vi "AB_1200_1100_Project_InteropAssembly_Info.vi"(7 "action":T3, 8 "error in (no error)":errorcluster, 10 "InteropAssebly info in":T2, 11 "Object In":T1) -> (0 "error out":errorcluster, 2 "InteropAssebly info out":T2, 3 "Object Out":T1)   [LabVIEW 2020]
uses:
  <vilib>/AppBuilder/RW_Project/AB_RW_Project_PropBag_Action.ctl
  <resource>/Framework/Providers/API/ItemRef.ctl
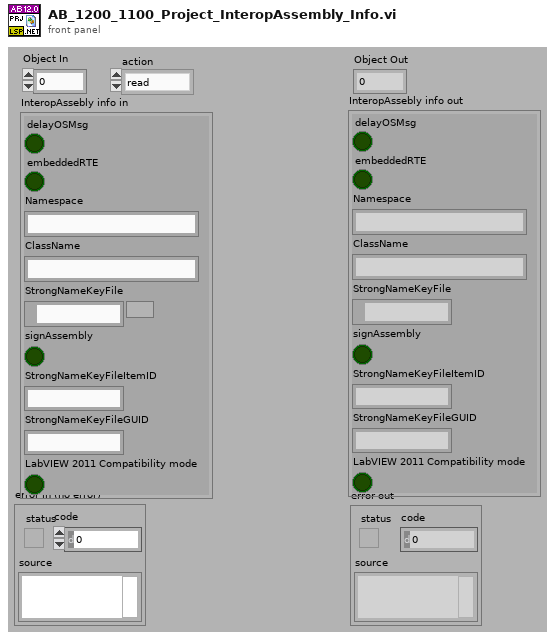
[diagram p1: front panel]
types:
  T1 = typedef "ItemRef.ctl" = u64
  T2 = cluster{"delayOSMsg":bool, "embeddedRTE":bool, "Namespace":string, "ClassName":string, "StrongNameKeyFile":path, "signAssembly":bool, "StrongNameKeyFileItemID":string, "StrongNameKeyFileGUID":string, "LabVIEW 2011 Compatibility mode":bool}
  T3 = typedef "AB_RW_Project_PropBag_Action.ctl" = enum16{"read", "write", "clear", "readPrevious", "writePrevious", "clearPrevious"}
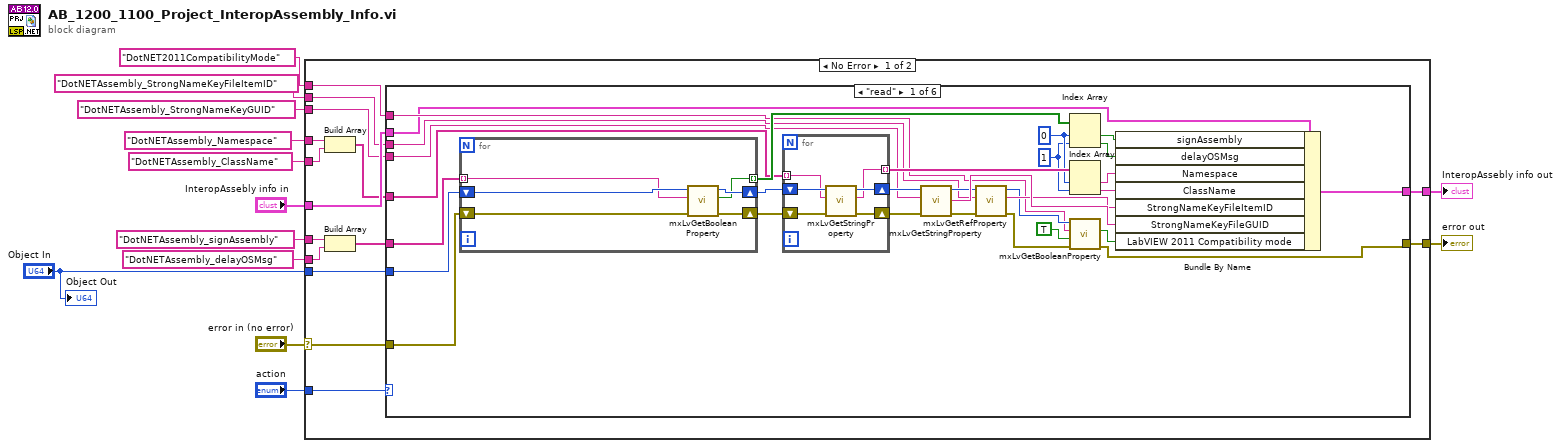
[diagram p0: block diagram]
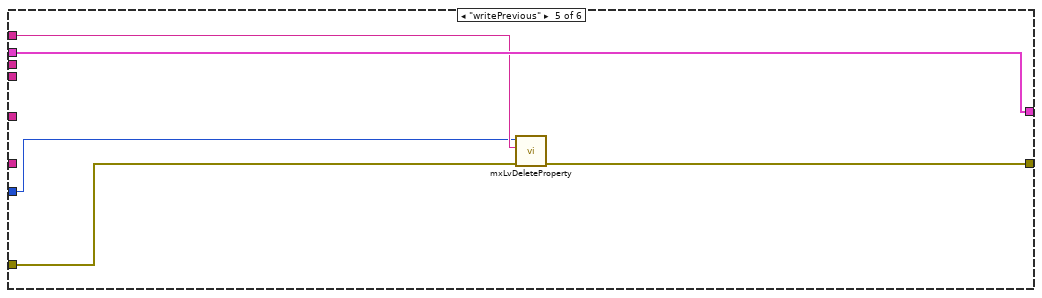
[diagram p5: hidden frame]
diagram:
  n1 = case shown="No Error" "error in (no error)" {
    selector: "error in (no error)" -> [w18 w85]
    tunnel: "Object In" -> [w27 _]
    tunnel: [w28 w84] -> w8
    tunnel: "InteropAssebly info in" -> [w26 w84]
    tunnel: "action" -> [w25 _]
    tunnel: "DotNETAssembly_Namespace" -> [w24 _]
    tunnel: "DotNETAssembly_ClassName" -> [w23 _]
    tunnel: "DotNETAssembly_StrongNameKeyGUID" -> [w21 _]
    tunnel: "DotNETAssembly_delayOSMsg" -> [w20 _]
    tunnel: [w17 w85] -> w4
    tunnel: "DotNETAssembly_StrongNameKeyFileItemID" -> [w16 _]
    tunnel: "DotNETAssembly_signAssembly" -> [w15 _]
    tunnel: "DotNET2011CompatibilityMode" -> [w14 _]
    frame No Error {
      n2 = Build Array(w24, w23) -> (w22:string[])
      n3 = Build Array(w15, w20) -> (w19:string[])
      n4 = case shown="\"read\"" w25 {
        tunnel: [w30 w72 w74 w76 w81 w83] -> w28
        tunnel: w27 -> [w37 _ _ _ w77 _]
        tunnel: w26 -> [w31 w72 w74 w76 w81 w83]
        tunnel: w22 -> [w35 _ _ _ _ _]
        tunnel: w21 -> [w34 _ _ _ _ _]
        tunnel: w19 -> [w36 _ _ _ _ _]
        tunnel: w18 -> [w38 w71 w73 w75 w79 w82]
        tunnel: [w29 w71 w73 w75 w78 w82] -> w17
        tunnel: w16 -> [w33 _ _ _ _ _]
        tunnel: w14 -> [w32 _ _ _ w80 _]
        frame "read" {
          w44 = 1 ("index")
          w52 = 0 ("index")
          n5 = for {
            shift-right: [w63] -> w55
            shift-left: w37 -> [w64]
            tunnel: w36 -> [w62] mode=indexing
            tunnel: [w61] -> w54 mode=indexing
            shift-right: [w59] -> w53
            shift-left: w38 -> [w60]
            n6 = call <resource>:"mxLvGetBooleanProperty.vi"("error in"=w60, "Tag"=w62, "Item"=w64) -> ("error out"=w59:errorcluster, "Value"=w61:bool, "Item"=w63:T1)  [unwired: 1 in, 5 out]
          }
          n7 = for {
            shift-right: [w69] -> w51
            shift-left: w55 -> [w70]
            tunnel: [w68] -> w58 mode=indexing
            tunnel: w35 -> [w67] mode=indexing
            shift-right: [w65] -> w50
            shift-left: w53 -> [w66]
            n8 = call <resource>:"mxLvGetStringProperty.vi"("Error In"=w66, "Tag"=w67, "Item"=w70) -> ("Error Out"=w65:errorcluster, "Value"=w68:string, "Item"=w69:T1)  [unwired: 6 out]
          }
          n9 = call <resource>:"mxLvGetStringProperty.vi"("Error In"=w50, "Tag"=w34, "Item"=w51) -> ("Error Out"=w47:errorcluster, "Value"=w49:string, "Item"=w46:T1)  [unwired: 6 out]
          n10 = call <resource>:"mxLvGetRefProperty.vi"("Error In"=w47, "Tag"=w33, "Item"=w46) -> ("Error Out"=w42:errorcluster, "Value"=w48:string, "Item"=w39:T1)  [unwired: 6 out]
          n11 = Index Array(array=w54, index #1=w52, index #2=w44) -> (element #1=w45:bool, element #2=w43:bool)
          n12 = Index Array(array=w58, index #1=w52, index #2=w44) -> (element #1=w57:string, element #2=w56:string)
          n13 = call <resource>:"mxLvGetBooleanProperty.vi"("error in"=w42, "Default Value (F)"=TRUE, "Tag"=w32, "Item"=w39) -> ("error out"=w29:errorcluster, "Value"=w41:bool)  [unwired: 6 out]
          n14 = Bundle By Name(cluster=w31, "signAssembly"=w45, "delayOSMsg"=w43, "Namespace"=w57, "ClassName"=w56, "StrongNameKeyFileItemID"=w48, "StrongNameKeyFileGUID"=w49, "LabVIEW 2011 Compatibility mode"=w41) -> (w30:T2)
        }
        frame "write" {
        }
        frame "clear" {
        }
        frame "readPrevious" {
        }
        frame "writePrevious" {
          n15 = call <resource>:"mxLvDeleteProperty.vi"("error in"=w79, "Tag"=w80, "Item"=w77) -> ("error out"=w78:errorcluster)  [unwired: 8 out]
        }
        frame "clearPrevious" {
        }
      }
    }
    frame Error {
    }
  }
  "error out" <- w4
  "InteropAssebly info out" <- w8
  "Object Out" <- "Object In"
